vi "Get Switch.vi"(8 "error in (no error)":errorcluster, 10 "Channel":u8=1, 11 "Queue in":T1) -> (0 "error out":errorcluster, 3 "Queue out":T1)   [LabVIEW 2019, in "Controller.lvlib"]
uses:
  Controller.lvlib
  Controller Message Queue.ctl
  Controller Message.ctl
  MDS Command.ctl
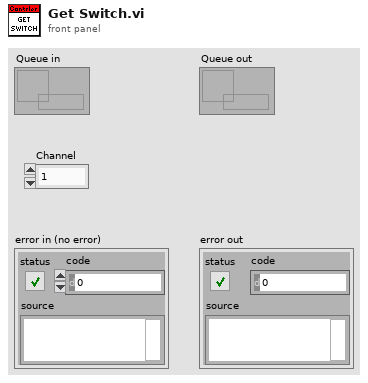
[diagram p1: front panel]
types:
  T1 = typedef "Controller.lvlib/Controller Message Queue.ctl" = refnum<queue>
  T2 = typedef "Controller.lvlib/Controller Message.ctl" = cluster{"MDS Command":T3, "Channel":u8, "Value":variant}
  T3 = typedef "Controller.lvlib/MDS Command.ctl" = enum16{"Idle", "Open", "Set VMode", "Set IMode", "Get Frequency", "Set Frequency", "Get Power", "Set Power (dBm)", "Set Power (%)", "Get Switch", "Switch Channel", "Store", "Wait for Prompt", "Wait for State", "Reset", "Error", "Close", "Stop"}
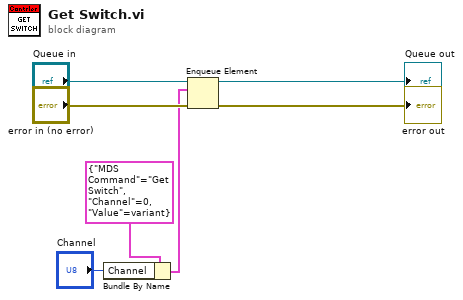
[diagram p0: block diagram]
diagram:
  n1 = Bundle By Name(cluster=T2 {"MDS Command"=enum."Get Switch", "Channel"=0, "Value"=variant} ("Controller Message"), "Channel"="Channel") -> (w2:T2)
  n2 = Enqueue Element(queue="Queue in", element=w2, error in (no error)="error in (no error)") -> (queue out=→"Queue out":T1, error out=→"error out":errorcluster)  [unwired: 1 in, 1 out]
